vi "Zero Phase Filter.vi"   [LabVIEW 2017, in "NI_AALBase.lvlib"]
doc: "Applies a zero phase filter to an input sequence <B>X</B>. Wire data to the <B>X</B> input to determine the polymorphic instance to use or manually select the instance."
uses:
  <vilib>/Analysis/NI_AALBase.lvlib
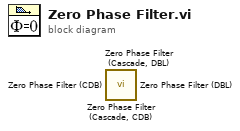
[diagram p0: block diagram]
diagram:
  n1 = call <vilib>:"Zero Phase Filter (Cascade, CDB).vi"() -> ()  [unwired: 10 in, 2 out]
  n2 = call <vilib>:"Zero Phase Filter (Cascade, DBL).vi"() -> ()  [unwired: 10 in, 2 out]
  n3 = call <vilib>:"Zero Phase Filter (CDB).vi"() -> ()  [unwired: 10 in, 2 out]
  n4 = call <vilib>:"Zero Phase Filter (DBL).vi"() -> ()  [unwired: 10 in, 2 out]
